vi "Rnm(r).vi"(4 "error in (no error)":errorcluster, 5 "n":i32, 6 "r":dbl, 7 "m":i32) -> (0 "error out":errorcluster, 2 "R nm (r)":dbl)   [LabVIEW 2020, in "Zernike Polynome.lvlib"]
doc: "This VI calculates the radial Zernike Polynomial coefficients."
uses:
  Zernike Polynome.lvlib
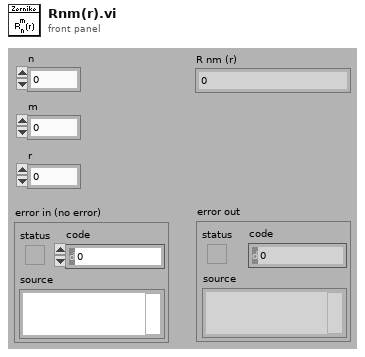
[diagram p1: front panel]
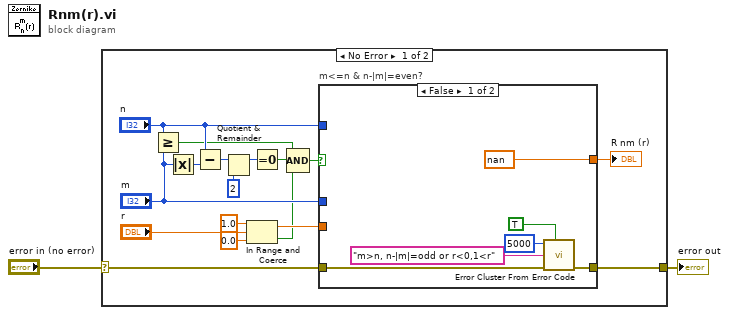
[diagram p0: block diagram]
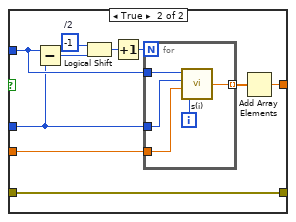
[diagram p2: hidden frame]
diagram:
  n1 = case shown="No Error" "error in (no error)" {
    selector: "error in (no error)" -> [w3 w41]
    tunnel: [w18 w41] -> w2
    frame No Error {
      n2 = Greater Or Equal?(x="n", y="m") -> (x >= y?=w9:bool)
      n3 = Absolute Value(x="m") -> (abs(x)=w14:i32)
      n4 = Subtract(x="n", y=w14) -> (x-y=w13:i32)
      n5 = Quotient & Remainder(x=w13, y=2) -> (x-y*floor(x/y)=w11:i32)  [unwired: 1 out]
      n6 = In Range and Coerce(upper limit=1.0, x="r", lower limit=0.0) -> (coerced(x)=w7:dbl, In Range?=w4:bool)
      n7 = Equal To 0?(x=w11) -> (x = 0?=w10:bool)
      n8 = Compound Arithmetic op=AND(w9, w10, w4) -> (w8:bool)
      n9 = case "m<=n & n-|m|=even?" shown="False" w8 {
        tunnel: "m" -> [_ w27]
        tunnel: "n" -> [_ w30]
        tunnel: w7 -> [_ w35]
        tunnel: w3 -> [w25 w34]
        tunnel: [w24 w34] -> w18
        tunnel: [nan w33] -> w16
        frame False {
          n10 = call <vilib>:"Error Cluster From Error Code.vi"("show call chain? (False)"=TRUE, "error in (no error)"=w25, "error message (\"\")"="m>n, n-|m|=odd or r<0,1<r" ("error message (\"\")"), "error code (0)"=5000) -> ("error out"=w24:errorcluster)  [unwired: 5 in]
        }
        frame True {
          w32 = -1  # /2
          n11 = Subtract(x=w30, y=w27) -> (x-y=w31:i32)
          n12 = Logical Shift(y=w32, x=w31) -> (x << y=w28:i32)
          n13 = Increment(x=w28) -> (x+1=w26:i32)
          n14 = for {
            N: w26 -> [_]
            tunnel: w35 -> [w40]
            tunnel: w30 -> [w37]
            tunnel: [w39] -> w29 mode=indexing
            tunnel: w27 -> [w38]
            i -> [w36]
            n15 = call "s(i).vi"("s"=w36, "r"=w40, "m"=w38, "n"=w37) -> ("R Sumand nm (r)"=w39:dbl)
          }
          n16 = Add Array Elements(numeric array=w29) -> (sum=w33:dbl)
        }
      }
      "R nm (r)" <- w16
    }
    frame Error {
    }
  }
  "error out" <- w2
